vi "All 1.vi"() -> ()   [LabVIEW 2022 SP3, in "Benchmark.lvlib"]
uses:
  Benchmark.lvlib
  Main/Scene/Scene.lvclass/Scene.ctl
  <vilib>/Utility/High Resolution Relative Seconds.vi
  Libraries/Utility/Convert Pixels To Picture.vi/d601d993-a776-4dc8-89c7-357d8398c88c.vi
  Libraries/Utility/Convert Pixels To Picture.vi/7816d0d6-8e4d-41a2-85ac-ed82f1435763.vi
  Main/Scene/Transform And Project.vi
  Main/Scene/Raster.vi
  Main/Scene/Update Object.vi
  Main/Scene/Update Transforms.vi
  Main/Scene/Transform And Project.vi/196e4586-e654-41ec-a3a4-43fea5068e8e.vi
  Libraries/3D/Calculate View Matrix.vi
  Main/Scene/Transform And Project.vi/a59a4b44-279f-4314-be75-e28f6a03f0ec.vi
  Main/Transform And Project Single Object.vi
  Libraries/3D/Sort Triangles.vi
  Main/Scene/Raster.vi/edb3f0c2-b950-4a44-8897-096d76b30880.vi
  Main/Scene/Raster.vi/76d78098-f527-454b-a08a-aac5a717328f.vi
  Libraries/3D/Raster.vi
  Main/Sub Vs/Create Y Rotation Matrix.vi
  Libraries/3D/Multiply Vector By Matrix.vi
  Libraries/3D/Point At.vi
  Libraries/3D/Matrix Quick Invert.vi
  Libraries/3D/Normal.vi
  Libraries/3D/Project And Illuminate Triangle.vi
  Libraries/3D/Apply View Matrix.vi
  Libraries/3D/Transform Triangle.vi
  Main/Sub Vs/Create Z Rotation Matrix.vi
  Main/Sub Vs/Create X Rotation Matrix.vi
  Main/Sub Vs/Create Translation Matrix.vi
  Libraries/3D/Check Raster Point In Range.vi
  Libraries/3D/Convert Point 2D (SGL) to Point 2D (I32).vi
  Libraries/Raster/Draw Triangle.vi
  Libraries/Raster/Draw Filled Triangle.vi
  Libraries/Raster/Clear Framebuffer.vi
  Libraries/3D/Degrees To Radians.vi
  Libraries/3D/Normalise Vector.vi
  Libraries/3D/Dot Product.vi
  Libraries/3D/Cross Product.vi
  Libraries/3D/Scale Point 3D (SGL) To Screen.vi
  Libraries/3D/Calculate Triangle Illumination.vi
  Libraries/Raster/Draw Line.vi
  Libraries/Raster/Draw Flat Bottom Filled Triangle.vi
  Libraries/Raster/Sort Points.vi
  Libraries/Raster/Draw Flat Top Filled Triangle.vi
  Libraries/Raster/Draw Line.vi/ce09c930-e75c-45b5-9de7-7d3097d91b09.vi
  Libraries/Raster/Draw Line.vi/8aa8c736-0805-475e-bbf3-9937bbefdeb4.vi
  Libraries/Raster/Draw Horizontal Line.vi
  Libraries/Raster/Draw Flat Bottom Filled Triangle.vi/c0c82237-b583-4fc1-b44f-40d02a28ecfd.vi
  Libraries/Raster/Draw Flat Bottom Filled Triangle.vi/53435b12-820c-4aea-aec4-7de16a894549.vi
  <vilib>/ptbypt/Probability & Statistics.llb/Mean PtByPt.vi
  <vilib>/Utility/colorconv.llb/Color to RGB.vi
  <vilib>/Utility/colorconv.llb/RGB to Color.vi
  <userlib>/_OpenG.lib/array/array.llb/Sort Array__ogtk.vi
  <userlib>/_OpenG.lib/array/array.llb/Sort 1D Array (SGL)__ogtk.vi
  <userlib>/_OpenG.lib/array/array.llb/Sort 1D Array (I32)__ogtk.vi
  <vilib>/picture/picture.llb/Draw Unflattened Pixmap.vi
  <vilib>/picture/picture.llb/Draw True-Color Pixmap.vi
  <vilib>/Analysis/NI_AALBase.lvlib
  Main/Scene/Scene.lvclass
  Libraries/Utility/Utility.lvlib
panel:
  out "2D Picture":picture
  out "Mean FPS":dbl format="%.1p"
  out "Std Dev":dbl format="%.1p"
  out "Mean":dbl format="%.1p"
  out "Histogram Graph":T1(graph)
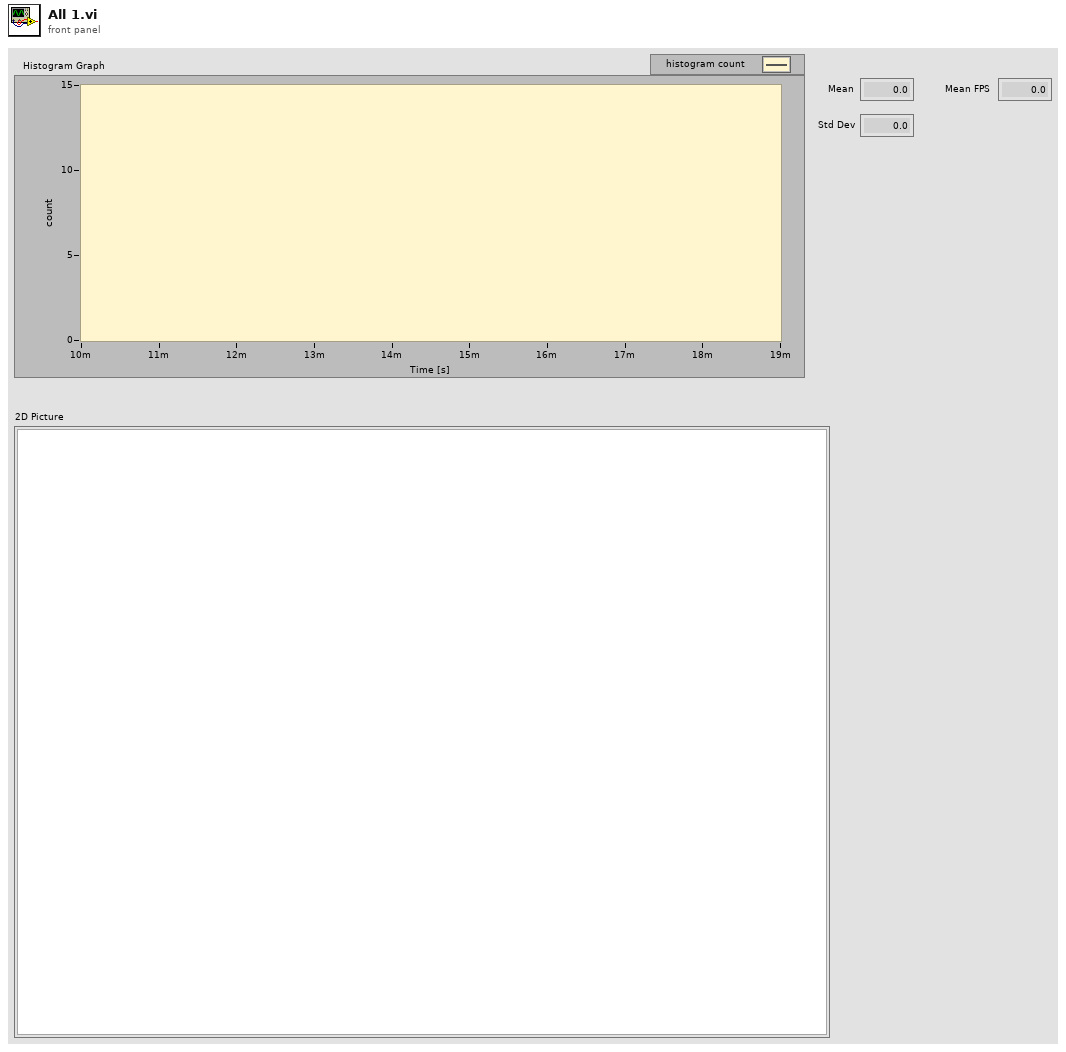
[diagram p1: front panel]
types:
  T1 = cluster{"X Values":dbl[], "Histogram: h(x)":i32[]}
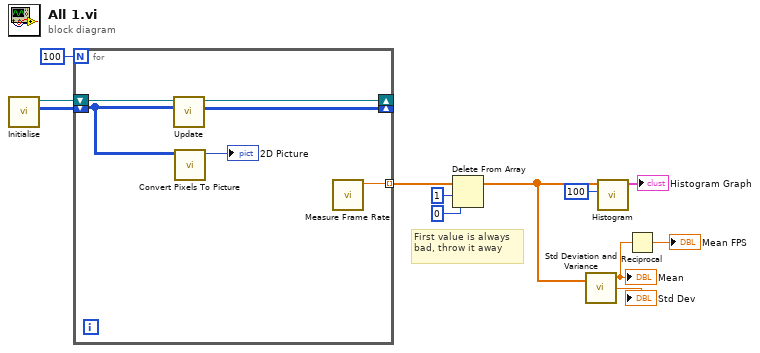
[diagram p0: block diagram]
diagram:
  # "First value is always bad, throw it away"
  n1 = call "Initialise.vi"() -> ("Pixel Data out"=w7:u32[][], "Scene out"=w8:refnum<class "Scene.lvclass">)  [unwired: 10 in]
  n2 = for {
    N: 100 -> [_]
    tunnel: [w13] -> w4 mode=indexing
    shift-right: [w15] -> _
    shift-left: w7 -> [w18]
    shift-right: [w14] -> _
    shift-left: w8 -> [w17]
    n3 = call "Update.vi"("Pixel Data in"=w18, "Scene in"=w17) -> ("Pixel Data out"=w15:u32[][], "Scene out"=w14:refnum<class "Scene.lvclass">)  [unwired: 8 in]
    n4 = call "Convert Pixels To Picture.vi"("Pixel Data in"=w18) -> ("2D Picture"=→"2D Picture":picture)  [unwired: 9 in, 1 out]
    n5 = call "Measure Frame Rate.vi"() -> ("Delta Time [s]"=w13:dbl)  [unwired: 10 in, 1 out]
  }
  n6 = Delete From Array(array=w4, length=1, index=0) -> (array with subset deleted=w3:dbl[])  [unwired: 1 out]
  n7 = call <vilib>:"Std Deviation and Variance.vi"("X"=w3) -> ("mean"=w6:dbl, "standard deviation"=→"Std Dev":dbl)  [unwired: 1 in, 1 out]
  "Mean" <- w6
  n8 = call <vilib>:"Histogram.vi"("intervals"=100, "X"=w3) -> ("Histogram Graph"=→"Histogram Graph":T1)  [unwired: 6 in, 3 out]
  n9 = Reciprocal(x=w6) -> (1/x=→"Mean FPS":dbl)
